vi "Arrays.vi"() -> ()   [LabVIEW 2013]
panel:
  in  "index":i32
  out "size(s)":i32
  out "element":dbl
  out "Array 5":dbl[](array[slide]) scale=0.0..10.0
  in  "Array 4":bool[](array[boolean])
  out "Array 3":bool[](array[boolean])
  in  "Array":dbl[](array[numeric])
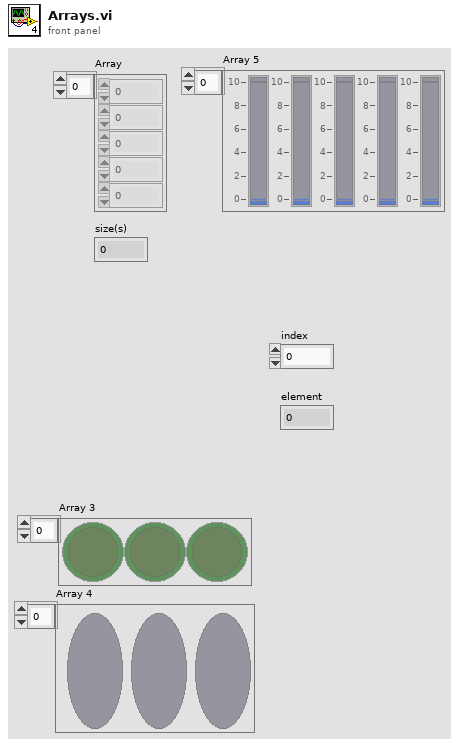
[diagram p1: front panel]
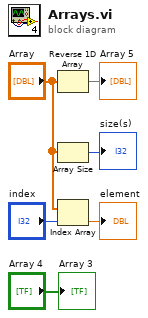
[diagram p0: block diagram]
diagram:
  n1 = Reverse 1D Array(array="Array") -> (reversed array=→"Array 5":dbl[])
  n2 = Array Size(array="Array") -> (size(s)=→"size(s)":i32)
  n3 = Index Array(array="Array", index="index") -> (element=→"element":dbl)
  "Array 3" <- "Array 4"
